vi "read_attributes.vi"(8 "error in (no error)":errorcluster caption="entrée d'erreur (pas d'erreur)", 11 "KMeans en entrée":refnum<class "KMeans.lvclass">) -> (0 "error out":errorcluster caption="sortie d'erreur", 2 "attributes":T1, 3 "KMeans en sortie":refnum<class "KMeans.lvclass">)   [LabVIEW 2020, in "KMeans.lvclass"]
uses:
  KMeans.lvclass
  Controls/kmeans_attributes.ctl
  KMeans.lvclass/KMeans.ctl
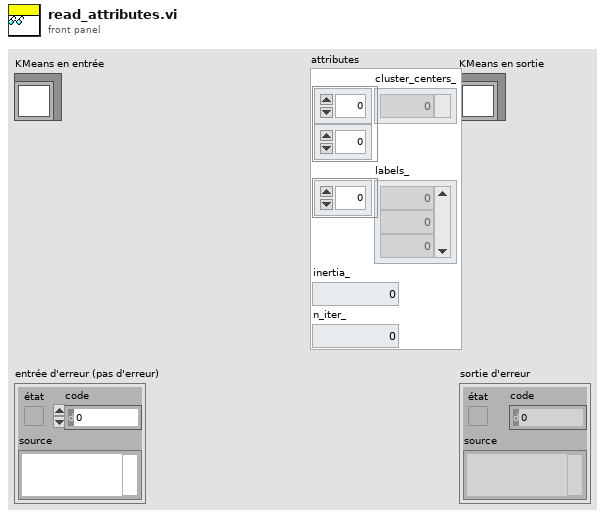
[diagram p1: front panel]
types:
  T1 = typedef "kmeans_attributes.ctl" = cluster{"cluster_centers_":dbl[][], "labels_":dbl[], "inertia_":dbl, "n_iter_":dbl}
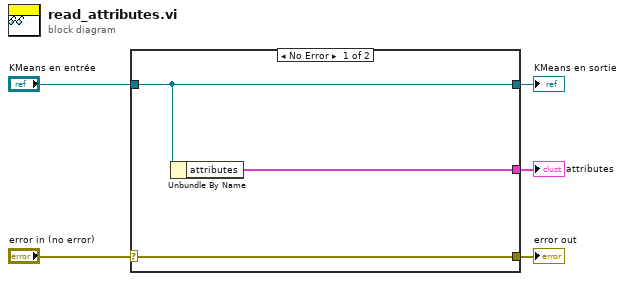
[diagram p0: block diagram]
diagram:
  n1 = case shown="No Error" "error in (no error)" {
    selector: "error in (no error)" -> [w8 w9]
    tunnel: [w8 w9] -> w4
    tunnel: [w7 w10] -> w2
    tunnel: "KMeans en entrée" -> [w7 w10]
    tunnel: [w6 _] -> w1
    frame No Error {
      n2 = Unbundle By Name(w7) -> ("attributes"=w6:T1)
    }
    frame Error {
    }
  }
  "error out" <- w4
  "KMeans en sortie" <- w2
  "attributes" <- w1
